vi "Communication - Reconnect eFGV.vi"(7 "eFGV States":T1, 8 "error in (no error)":errorcluster, 11 "Reconnect In":string) -> (0 "error out":errorcluster, 2 "Reconnect Ref":refnum<user-event>, 3 "Reconnect Out":string)   [LabVIEW 2019]
doc: "event FGV where it will trigger to stop all the process in the program"
uses:
  Controls/eFGV States.ctl
  <vilib>/event_ctls.llb/usereventprio.ctl
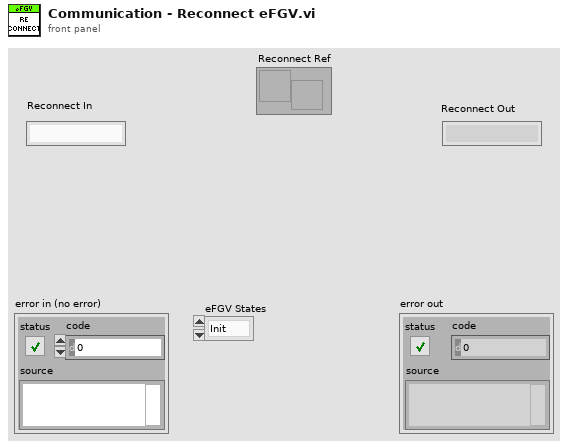
[diagram p1: front panel]
types:
  T1 = typedef "eFGV States.ctl" = enum16{"Init", "Read", "Write", "Exit"}
  T2 = typedef "usereventprio.ctl" = enum32{"high priority", "normal priority"}
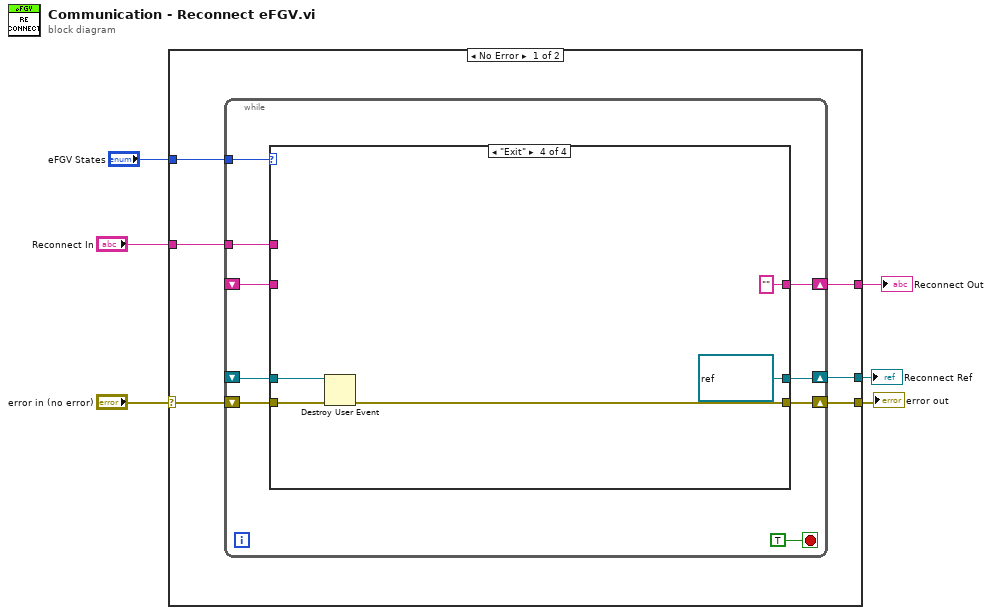
[diagram p0: block diagram]
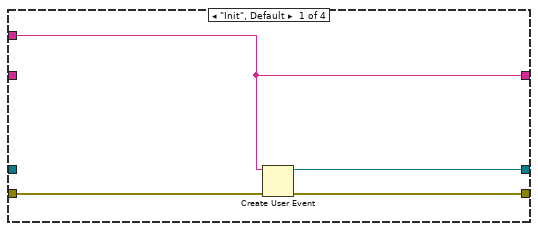
[diagram p2: hidden frame]
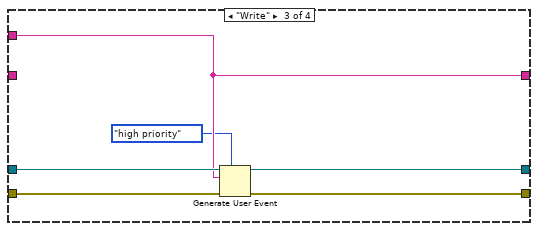
[diagram p4: hidden frame]
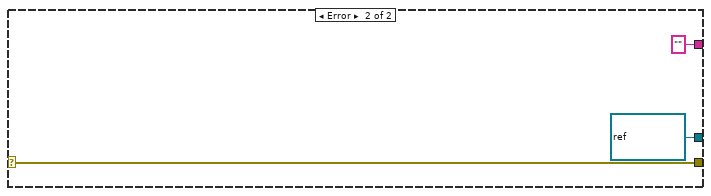
[diagram p5: hidden frame]
diagram:
  n1 = case shown="No Error" "error in (no error)" {
    selector: "error in (no error)" -> [w11 w42]
    tunnel: "eFGV States" -> [w12 _]
    tunnel: "Reconnect In" -> [w10 _]
    tunnel: [w9 w42] -> w3
    tunnel: [w8 "" ("Reconnect In")] -> w2
    tunnel: [w7 refnum<user-event> refnum ("Reconnect In")] -> w1
    frame No Error {
      n2 = while {
        tunnel: w12 -> [w20]
        shift-right: [w17] -> w9
        shift-left: w11 -> [w19]
        tunnel: w10 -> [w18]
        shift-right: [w16] -> w8
        shift-left: _ -> [w15]
        shift-right: [w14] -> w7
        shift-left: _ -> [w13]
        stop <- TRUE stop-if-true
        n3 = case shown="\"Exit\"" w20 {
          tunnel: w19 -> [w25 w27 w32 w39]
          tunnel: w18 -> [w23 _ w31 _]
          tunnel: [w24 w27 w33 w37] -> w17
          tunnel: [w23 w28 w31 "" ("Reconnect In")] -> w16
          tunnel: w15 -> [_ w28 _ _]
          tunnel: w13 -> [_ w26 w34 w38]
          tunnel: [w22 w26 w29 refnum<user-event> refnum ("Reconnect In")] -> w14
          frame "Init", Default {
            n4 = Create User Event(user event datatype=w23, error in=w25) -> (user event=w22:refnum<user-event>, error out=w24:errorcluster)
          }
          frame "Read" {
          }
          frame "Write" {
            n5 = Generate User Event(priority (normal)=usereventprio."high priority", user event=w34, event data cluster=w31, error in=w32) -> (user event out=w29:refnum<user-event>, error out=w33:errorcluster)
          }
          frame "Exit" {
            n6 = Destroy User Event(user event=w38, error in=w39) -> (error out=w37:errorcluster)
          }
        }
      }
    }
    frame Error {
    }
  }
  "error out" <- w3
  "Reconnect Out" <- w2
  "Reconnect Ref" <- w1
